vi "Set PluginCore RefreshStatistics Response.vi"(7 "Streaming? (F)":bool, 8 "error in (no error)":errorcluster, 10 "Message Data":T1, 11 "gRPCid in":T3) -> (0 "error out":errorcluster)   [LabVIEW 2021, in "CIFCorePlugin_server.lvlib" / "PluginCore.lvclass"]
uses:
  PluginCore.lvclass
  <vilib>/gRPC/LabVIEW gRPC Library/Shared/grpcId.ctl
  <vilib>/gRPC/gRPC Server and Client Template [2]/Server Template/RPC Messages/Set package_templatemessage.vi/dcc74a39-081a-4bdd-860b-8ed792803c96.vi
  <vilib>/gRPC/gRPC Server and Client Template [2]/Server Template/RPC Messages/Set package_templatemessage.vi/c8cd2a7d-3f0e-47f4-bd6c-d8bf1e02ce4e.vi
  <vilib>/gRPC/LabVIEW gRPC Library/Shared/TranslateGrpcError.vi
  <vilib>/gRPC/LabVIEW gRPC Library/Server API/Server/Get Server DLL Path.vi
  <vilib>/Utility/error.llb/Error Cluster From Error Code.vi
  <vilib>/gRPC/LabVIEW gRPC Library/Server API/Message Requests/Complete Call.vi
  PluginCore.lvclass/PluginCore.ctl
  CIFCorePlugin_server.lvlib
  <vilib>/gRPC/LabVIEW gRPC Library/grpc-lvsupport-release.lvlib
  RPC Messages/cif_common_Status.ctl
  RPC Messages/cif_plugincore_RefreshStatisticsResponse.ctl
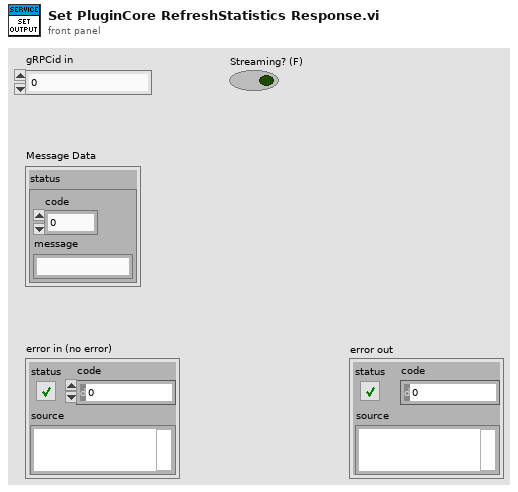
[diagram p1: front panel]
types:
  T1 = typedef "CIFCorePlugin_server.lvlib/cif_plugincore_RefreshStatisticsResponse.ctl" = cluster{"status":T2}
  T2 = typedef "CIFCorePlugin_server.lvlib/cif_common_Status.ctl" = cluster{"code":i32, "message":string}
  T3 = typedef "grpc-lvsupport-release.lvlib/grpcId.ctl" = u64
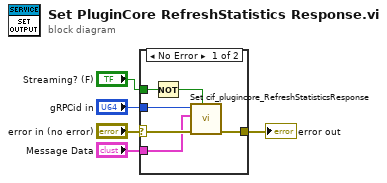
[diagram p0: block diagram]
diagram:
  n1 = case shown="No Error" "error in (no error)" {
    selector: "error in (no error)" -> [w11 w12]
    tunnel: [w9 w12] -> w4
    tunnel: "gRPCid in" -> [w10 _]
    tunnel: "Message Data" -> [w8 _]
    tunnel: "Streaming? (F)" -> [w7 _]
    frame No Error {
      n2 = Not(x=w7) -> (.not. x?=w6:bool)
      n3 = call "Set cif_plugincore_RefreshStatisticsResponse.vi"("Complete Call (T)"=w6, "error in (no error)"=w11, "package_templatemessage"=w8, "gRPCid"=w10) -> ("error out"=w9:errorcluster)  [unwired: 7 in]
    }
    frame Error {
    }
  }
  "error out" <- w4
